vi "Retrieve Root Actor.vi"(8 "error in (no error)":errorcluster, 11 "Target Store in":refnum<class "Target Store.lvclass">) -> (0 "error out":errorcluster, 1 "valid?":bool, 2 "Root Actor":path, 3 "Target Store out":refnum<class "Target Store.lvclass">)   [LabVIEW 2023, in "Add Actor.lvlib" / "Target Store.lvclass"]
uses:
  Target Store.lvclass
  Target Store.lvclass/Target Store.ctl
  AFPP Shared/Constants.vi
  AFPP Shared/AFPP Shared.lvlib
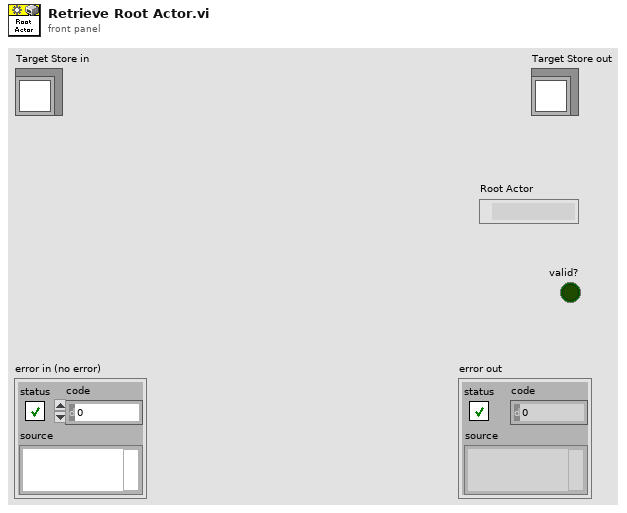
[diagram p1: front panel]
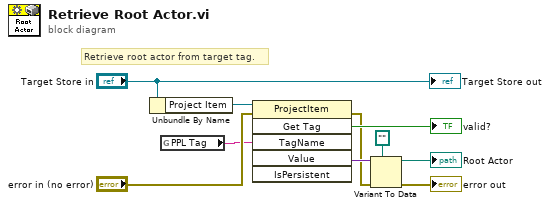
[diagram p0: block diagram]
diagram:
  # "Retrieve root actor from target tag."
  n1 = Unbundle By Name("Target Store in") -> ("Project Item"=w6:refnum<vi>)
  n2 = global read "Constants.vi" "PPL Tag"() -> (w2:string)
  n3 = invoke class="ProjectItem" method="Get Tag"(reference=w6, error in="error in (no error)", "TagName"=w2) -> (error out=w3:errorcluster, "GetTag"=→"valid?":bool, "Value"=w5:variant)  [unwired: 3 in, 3 out]
  n4 = Variant To Data(error in=w3, type=path "", Variant=w5) -> (data=→"Root Actor":path, error out=→"error out":errorcluster)
  "Target Store out" <- "Target Store in"
